vi "Poll Syringe-Capillary Valve Control.vi"(8 "error in (no error)":errorcluster, 11 "Capillary Line in":refnum<class "Capillary Line.lvclass">) -> ()   [LabVIEW 2015, in "cRIO-Carbondioxide.lvlib" / "CO2-Actor.lvlib" / "Capillary Line.lvclass"]
uses:
  Capillary Line.lvclass
  Capillary Line.lvclass/Capillary Line.ctl
  <vilib>/ActorFramework/Actor/Actor.lvclass/Actor.ctl
  <vilib>/ActorFramework/Message Enqueuer/Message Enqueuer.lvclass/Message Enqueuer.ctl
  Capillary Line Messages/Set Capillary Valve Msg/Set Capillary Valve Msg.lvclass/Set Capillary Valve Msg.ctl
  <vilib>/ActorFramework/Actor/Read Self Enqueuer.vi
  <vilib>/ActorFramework/Message Enqueuer/Enqueue.vi
  <vilib>/ActorFramework/Message Enqueuer/Init from Existing Queue.vi
  <vilib>/ActorFramework/Message Priority Queue/Priority Enqueue.vi
  <vilib>/ActorFramework/Actor/Actor.lvclass
  <vilib>/ActorFramework/Message Enqueuer/Message Enqueuer.lvclass
  Capillary Line Messages/Set Capillary Valve Msg/Set Capillary Valve Msg.lvclass
  cRIO-CO2/cRIO-CO2.lvclass
  CO2 Actor/CO2 Actor.lvclass
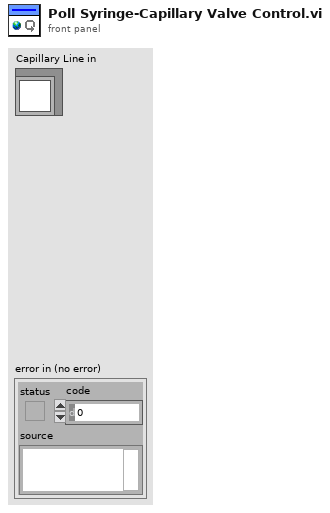
[diagram p1: front panel]
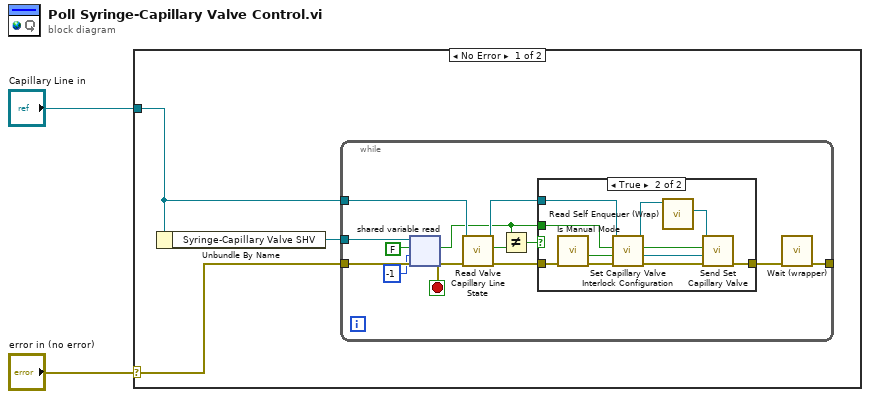
[diagram p0: block diagram]
diagram:
  n1 = case shown="No Error" "error in (no error)" {
    selector: "error in (no error)" -> [w3 _]
    tunnel: "Capillary Line in" -> [w4 _]
    frame No Error {
      n2 = Unbundle By Name(w4) -> ("Syringe-Capillary Valve SHV"=w5:refnum<k21>)
      n3 = while {
        tunnel: w5 -> [w18]
        tunnel: w3 -> [w17]
        tunnel: w4 -> [w12]
        tunnel: [w6] -> _
        stop <- w14 stop-if-true
        n4 = shared-variable-read(w18, w17, FALSE, -1 ("timeout ms")) -> (w14:errorcluster, w9:bool)  [unwired: 3 out]
        n5 = call "Read Valve Capillary Line State.vi"("error in (no error)"=w14, "Capillary Line in"=w12) -> ("error out"=w13:errorcluster, "Open?"=w10:bool, "Capillary Line out"=w11:refnum<class "Capillary Line.lvclass">)  [unwired: 5 in, 2 out]
        n6 = Not Equal?(x=w9, y=w10) -> (x != y?=w8:bool)
        n7 = case shown="True" w8 {
          tunnel: [w19 w29] -> w7
          tunnel: w13 -> [w19 w22]
          tunnel: w11 -> [_ w21]
          tunnel: w9 -> [_ w20]
          frame False {
          }
          frame True {
            n8 = call "Is Manual Mode.vi"("error in (no error)"=w22) -> ("error out"=w28:errorcluster, "Manual Mode?"=w23:bool)  [unwired: 9 in]
            n9 = call "Set Capillary Valve Interlock Configuration.vi"("error in (no error)"=w28, "Manual Mode (False)"=w23, "Open? (False)"=w20, "Capillary Line in"=w21) -> ("error out"=w26:errorcluster, "Interlock Chain"=w25:refnum<class "Interlock Chain.lvclass">, "Open? (False)"=w24:bool, "Capillary Line out"=w27:refnum<class "Capillary Line.lvclass">)  [unwired: 4 in]
            n10 = call "Read Self Enqueuer (Wrap).vi"("CO2 Actor in"=w27) -> ("Actor Framework:Message Enqueuer"=w30:refnum<class "Message Enqueuer.lvclass">)  [unwired: 9 in, 1 out]
            n11 = call "Send Set Capillary Valve.vi"("error in (no error)"=w26, "Interlock Chain.lvclass"=w25, "Open? (False)"=w24, "Message Enqueuer"=w30) -> ("error out"=w29:errorcluster)  [unwired: 6 in, 1 out]
          }
        }
        n12 = call "Wait (wrapper).vi"("error in (no error)"=w7) -> ("error out"=w6:errorcluster)  [unwired: 10 in]
      }
    }
    frame Error {
    }
  }
